vi "tarea2-1.vi"(4 "D":bool, 5 "C":bool, 6 "B":bool, 7 "A":bool) -> (0 "Z":bool, 1 "Y":bool, 2 "X":bool, 3 "W":bool)   [LabVIEW 2016]
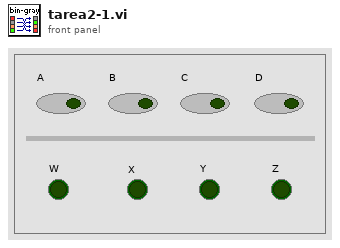
[diagram p1: front panel]
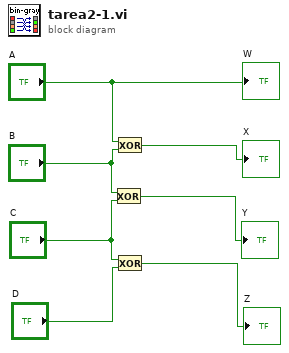
[diagram p0: block diagram]
diagram:
  n1 = Exclusive Or(1:"C", 2:"B") -> (0:→"Y":bool)
  n2 = Exclusive Or(1:"B", 2:"A") -> (0:→"X":bool)
  n3 = Exclusive Or(1:"D", 2:"C") -> (0:→"Z":bool)
  "W" <- "A"
